vi "setControlDisplayState.vi"(7 "Disabled":T1(ring), 8 "error in (no error)":errorcluster, 11 "Control Refs In":refnum<vi>[](array[refnum])) -> (0 "error out":errorcluster, 3 "Control Refs Out":refnum<vi>[](array[refnum]))   [LabVIEW 2011]
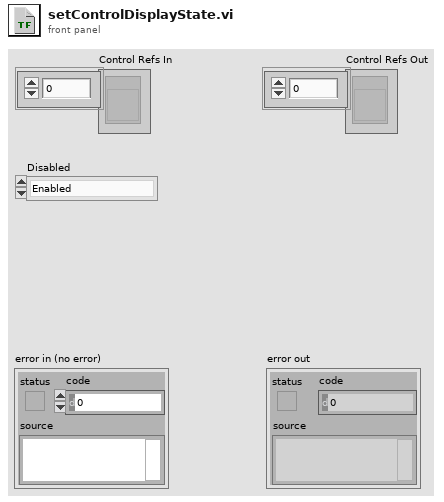
[diagram p1: front panel]
types:
  T1 = enum8{"Enabled", "Disabled", "Disabled and Grayed Out"}
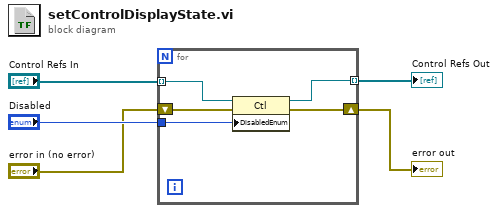
[diagram p0: block diagram]
diagram:
  n1 = for {
    tunnel: "Disabled" -> [w10]
    tunnel: "Control Refs In" -> [w9] mode=indexing
    tunnel: [w8] -> w3 mode=indexing
    shift-right: [w6] -> w1
    shift-left: "error in (no error)" -> [w7]
    n2 = property class="Ctl"(reference=w9, error in=w7, "DisabledEnum"=w10) -> (reference out=w8:refnum<vi>, error out=w6:errorcluster)
  }
  "Control Refs Out" <- w3
  "error out" <- w1
